vi "UpdateRef.vi"(8 "error in (no error)":errorcluster, 11 "Menu in":refnum<class "MGI_Menu.lvclass">) -> (0 "error out":errorcluster, 3 "Menu out":refnum<class "MGI_Menu.lvclass">)   [LabVIEW 2016, in "MGI_Menu.lvclass"]
doc: "Authored by Derek E. Trepanier\nsupport@mooregoodideas.com\nwww.mooregoodideas.com\n\nCopyright (c) 2012, Moore Good Ideas, Inc.\n\nAll rights reserved.\n\nRedistribution and use in source and binary forms, with or without modification, are permitted provided that the following conditions are met:\n\n * Redistributions of source code must retain the above copyright notice, this list of conditions and the following disclaimer.\n * Redistributions in binary form must reproduce the above copyright notice, this list of conditions and the following disclaimer in the documentation and/or other materials provided with the distribution.\n * Neither the name of Moore Good Ideas, Inc. nor the names of its contributors may be used to endorse or promote products derived from this software without specific prior written permission.\n\nTHIS SOFTWARE IS PROVIDED BY THE COPYRIGHT HOLDERS AND CONTRIBUTORS \"AS IS\" AND ANY EXPRESS OR IMPLIED WARRANTIES, INCLUDING, BUT NOT LIMITED TO, THE IMPLIED WARRANTIES OF MERCHANTABILITY AND FITNESS FOR A PARTICULAR PURPOSE ARE DISCLAIMED. IN NO EVENT SHALL THE COPYRIGHT OWNER OR CONTRIBUTORS BE LIABLE FOR ANY DIRECT, INDIRECT, INCIDENTAL, SPECIAL, EXEMPLARY, OR CONSEQUENTIAL DAMAGES (INCLUDING, BUT NOT LIMITED TO, PROCUREMENT OF SUBSTITUTE GOODS OR SERVICES; LOSS OF USE, DATA, OR PROFITS; OR BUSINESS INTERRUPTION) HOWEVER CAUSED AND ON ANY THEORY OF LIABILITY, WHETHER IN CONTRACT, STRICT LIABILITY, OR TORT (INCLUDING NEGLIGENCE OR OTHERWISE) ARISING IN ANY WAY OUT OF THE USE OF THIS SOFTWARE, EVEN IF ADVISED OF THE POSSIBILITY OF SUCH DAMAGE."
uses:
  <userlib>/_MGI/Menu Building/MenuTypes/MGI_Menu.lvclass
  <userlib>/_MGI/Menu Building/MenuTypes/MGI_Menu.lvclass/MGI_Menu.ctl
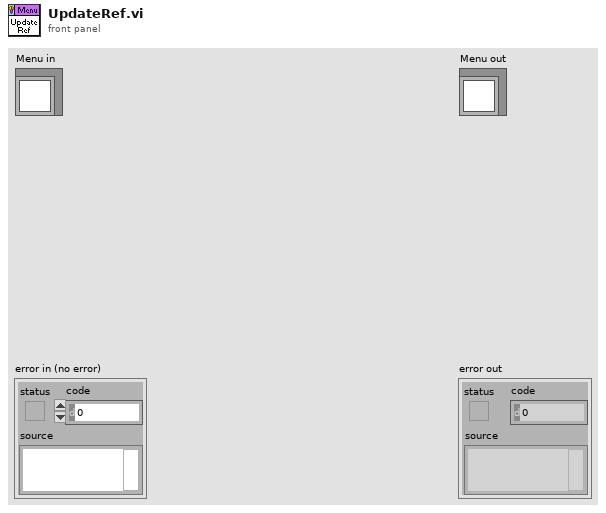
[diagram p1: front panel]
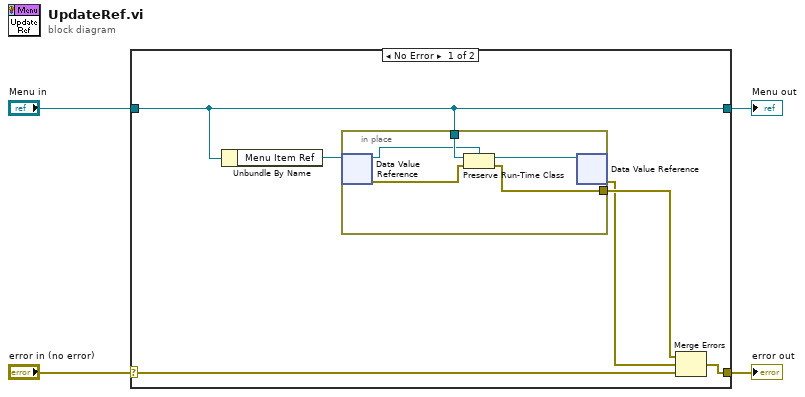
[diagram p0: block diagram]
diagram:
  n1 = case shown="No Error" "error in (no error)" {
    selector: "error in (no error)" -> [w6 w17]
    tunnel: [w5 w17] -> w3
    tunnel: [w9 w16] -> w1
    tunnel: "Menu in" -> [w9 w16]
    frame No Error {
      n2 = Unbundle By Name(w9) -> ("Menu Item Ref"=w10:refnum<data-value>)
      n3 = in-place {
        in-place-border: w9 -> [w15]
        in-place-border: [w11] -> w8
        n4 = in-place-dvr #1(w10) -> (w13:refnum<class>, w12:errorcluster)
        n5 = Preserve Run-Time Class(object in=w15, error in=w12, 2:w13) -> (object out=w14:refnum<class>, error out=w11:errorcluster)
        n6 = in-place-dvr #1(w14) -> (w7:errorcluster)  [unwired: 1 out]
      }
      n7 = Merge Errors(w8, w7, w6) -> (w5:errorcluster)
    }
    frame Error {
    }
  }
  "error out" <- w3
  "Menu out" <- w1
